vi "Write UI State.vi"(8 "error in (no error)":errorcluster, 10 "UI State":string, 11 "Update UI Status in":refnum<class "Update UI Status.lvclass">) -> (0 "error out":errorcluster, 3 "Update UI Status out":refnum<class "Update UI Status.lvclass">)   [LabVIEW 2019, in "User Interface Process.lvlib" / "Update UI Status.lvclass"]
uses:
  Update UI Status.lvclass
  Update UI Status.lvclass/Update UI Status.ctl
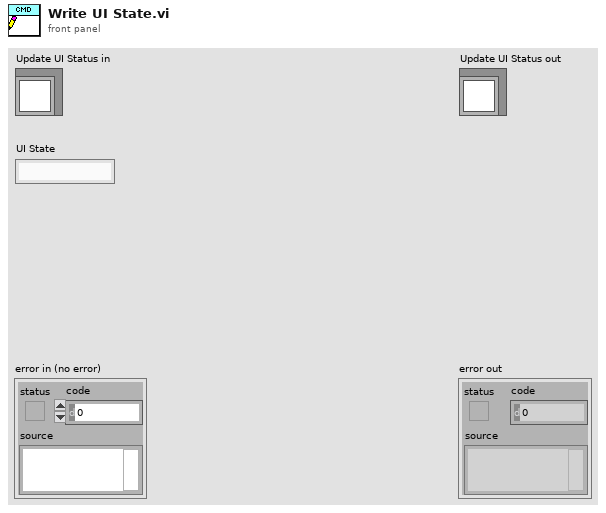
[diagram p1: front panel]
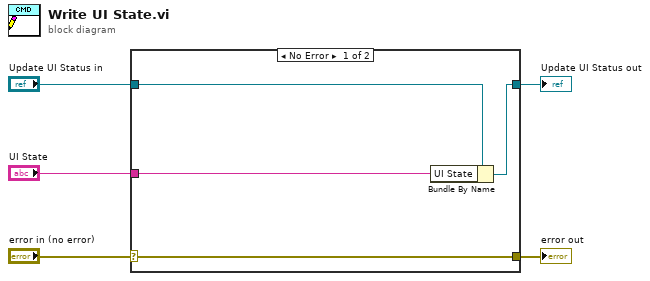
[diagram p0: block diagram]
diagram:
  n1 = case shown="No Error" "error in (no error)" {
    selector: "error in (no error)" -> [w9 w10]
    tunnel: [w9 w10] -> w4
    tunnel: [w7 w11] -> w2
    tunnel: "Update UI Status in" -> [w8 w11]
    tunnel: "UI State" -> [w6 _]
    frame No Error {
      n2 = Bundle By Name(cluster=w8, "UI State"=w6) -> (w7:refnum<class "Update UI Status.lvclass">)
    }
    frame Error {
    }
  }
  "error out" <- w4
  "Update UI Status out" <- w2
